vi "Register Cancel.vi"(8 "error in (no error)":errorcluster, 9 "Data Message":refnum<class "Data Message.lvclass">, 10 "View Enqueuer":refnum<class "Message Enqueuer.lvclass">, 11 "Print View in":refnum<class "Print View.lvclass">) -> (0 "error out":errorcluster, 3 "Print View out":refnum<class "Print View.lvclass">)   [LabVIEW 2015, in "Print View.lvlib" / "Print View.lvclass"]
uses:
  Print View.lvclass
  <vilib>/ActorFramework/Message Enqueuer/Message Enqueuer.lvclass
  <vilib>/ActorFrameworkObserver/Data Message/Data Message.lvclass
  Print View.lvclass/Print View.ctl
  <vilib>/ActorFrameworkObserver/Actor Register/Actor Register.lvclass
panel:
  # "NOTICE -- YOU MUST LEAVE THIS NOTICE IN PLACE.\n\nCopyright (c) 2015, LIANG LIU Shawn.Liu.cn@gmail.com\nAll rights reserved.\n\nRedistribution and use in source and binary forms, with or without modification, are permitted provided that the following conditions are met:\n-Redistributions of source code must retain the above copyright notice, this list of conditions and the following disclaimer.\n-Redistributions in binary form must reproduce the above copyright notice, this list of conditions and the following disclaimer in the documentation and/or other materials provided with the distribution.\n-Neither the name of the eLp nor the names of its contributors may be used to endorse or promote products derived from this software without specific prior written permission.\n\nTHIS SOFTWARE IS PROVIDED BY THE COPYRIGHT HOLDERS AND CONTRIBUTORS \"AS IS\" AND ANY EXPRESS OR IMPLIED WARRANTIES, INCLUDING, BUT NOT LIMITED TO, THE IMPLIED WARRANTIES OF MERCHANTABILITY AND FITNESS FOR A PARTICULAR PURPOSE ARE DISCLAIMED. IN NO EVENT SHALL THE COPYRIGHT HOLDER OR CONTRIBUTORS BE LIABLE FOR ANY DIRECT, INDIRECT, INCIDENTAL, SPECIAL, EXEMPLARY, OR CONSEQUENTIAL DAMAGES (INCLUDING, BUT NOT LIMITED TO, PROCUREMENT OF SUBSTITUTE GOODS OR SERVICES; LOSS OF USE, DATA, OR PROFITS; OR BUSINESS INTERRUPTION) HOWEVER CAUSED AND ON ANY THEORY OF LIABILITY, WHETHER IN CONTRACT, STRICT LIABILITY, OR TORT (INCLUDING NEGLIGENCE OR OTHERWISE) ARISING IN ANY WAY OUT OF THE USE OF THIS SOFTWARE, EVEN IF ADVISED OF THE POSSIBILITY OF SUCH DAMAGE."
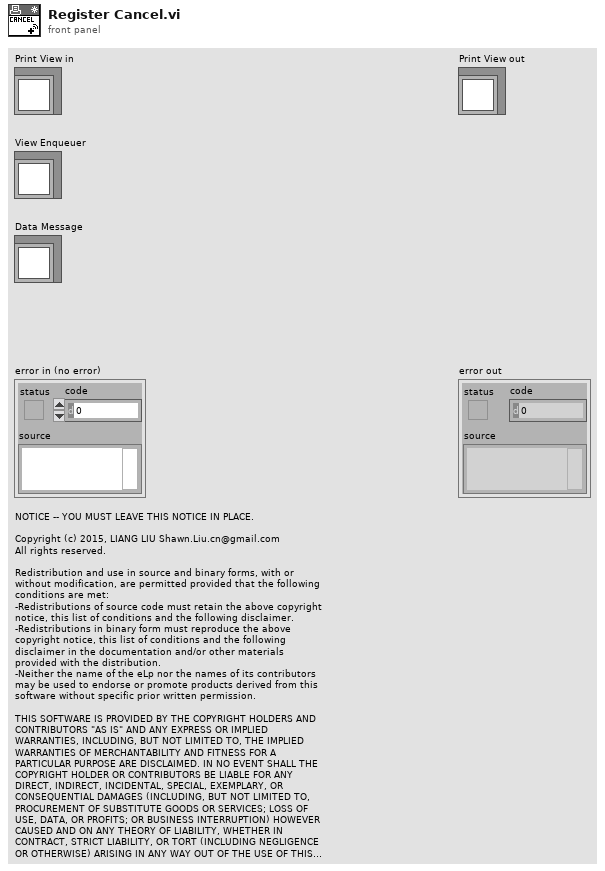
[diagram p1: front panel]
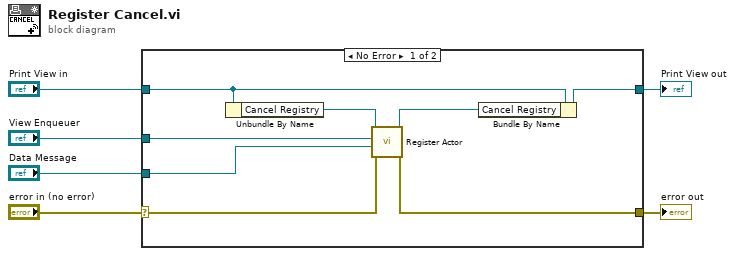
[diagram p0: block diagram]
diagram:
  n1 = case shown="No Error" "error in (no error)" {
    selector: "error in (no error)" -> [w12 w16]
    tunnel: "View Enqueuer" -> [w14 _]
    tunnel: "Print View in" -> [w8 w15]
    tunnel: "Data Message" -> [w13 _]
    tunnel: [w7 w15] -> w2
    tunnel: [w11 w16] -> w1
    frame No Error {
      n2 = Unbundle By Name(w8) -> ("Cancel Registry"=w10:refnum<class "Actor Register.lvclass">)
      n3 = call <vilib>:"Register Actor.vi"("error in (no error)"=w12, "Data Message"=w13, "Actor Enqueuer"=w14, "Actor Register in"=w10) -> ("error out"=w11:errorcluster, "Actor Register out"=w9:refnum<class "Actor Register.lvclass">)  [unwired: 6 in]
      n4 = Bundle By Name(cluster=w8, "Cancel Registry"=w9) -> (w7:refnum<class "Print View.lvclass">)
    }
    frame Error {
    }
  }
  "error out" <- w1
  "Print View out" <- w2
